vi "readFromXML.vi"(8 "error in (no error)":errorcluster, 10 "XML in":string, 11 "ScienceTargetAbsorbOffset in":refnum<class "ScienceTargetAbsorbOffset.lvclass">) -> (0 "error out":errorcluster, 3 "ScienceTargetAbsorbOffset out":refnum<class "ScienceTargetAbsorbOffset.lvclass">)   [LabVIEW 2014, in "TCSDataDefinitions.lvlib" / "TCSCommand.lvlib" / "OffsetCommands.lvlib" / "ScienceTargetAbsorbOffset.lvclass"]
uses:
  ScienceTargetAbsorbOffset.lvclass
  AbsorbOffset/AbsorbOffset.lvclass
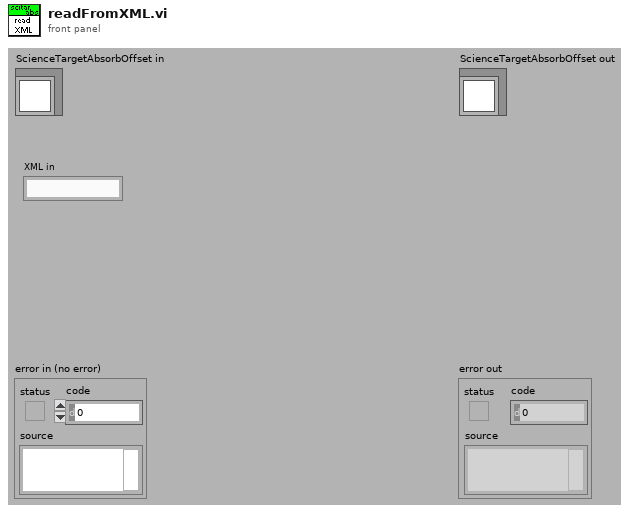
[diagram p1: front panel]
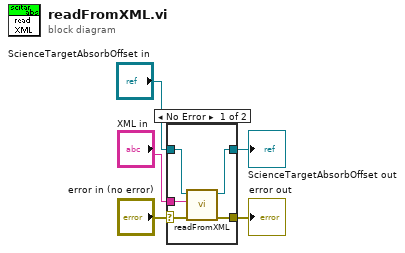
[diagram p0: block diagram]
diagram:
  n1 = case shown="No Error" "error in (no error)" {
    selector: "error in (no error)" -> [w8 w12]
    tunnel: [w7 w12] -> w4
    tunnel: [w9 w11] -> w2
    tunnel: "ScienceTargetAbsorbOffset in" -> [w10 w11]
    tunnel: "XML in" -> [w6 _]
    frame No Error {
      n2 = call-parent "readFromXML.vi"("error in (no error)"=w8, "XML in"=w6, "AbsorbOffset in"=w10) -> ("error out"=w7:errorcluster, "AbsorbOffset out"=w9:refnum<class "ScienceTargetAbsorbOffset.lvclass">)  [unwired: 7 out]
    }
    frame Error {
    }
  }
  "error out" <- w4
  "ScienceTargetAbsorbOffset out" <- w2
